vi "OFDM TX.vi"(1 "Samples/Symbol":i32, 2 "Waveform":waveform(cdb)) -> (0 "TX Signal":waveform(cdb))   [LabVIEW 2018]
panel:
  out "size(s)":i32
  out "Waveform w/ Center Freq":dbl[](graph)
  # "Note: Amplitude spikes at start/end of a symbol, reason unknown.\nMay be addressed with QAM Windowing?"
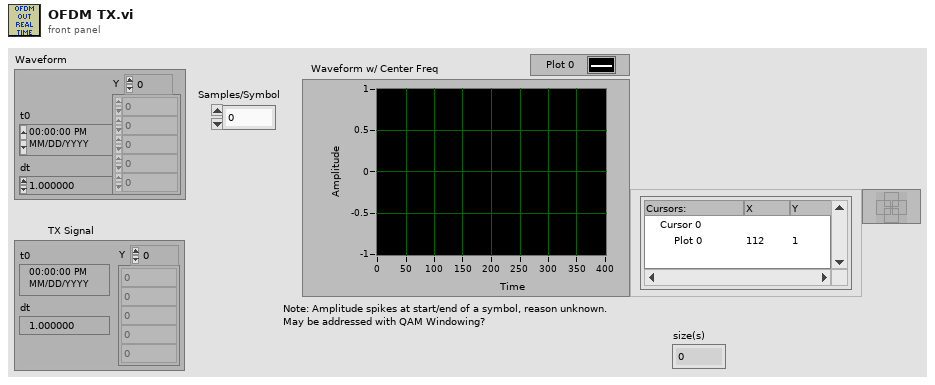
[diagram p1: front panel]
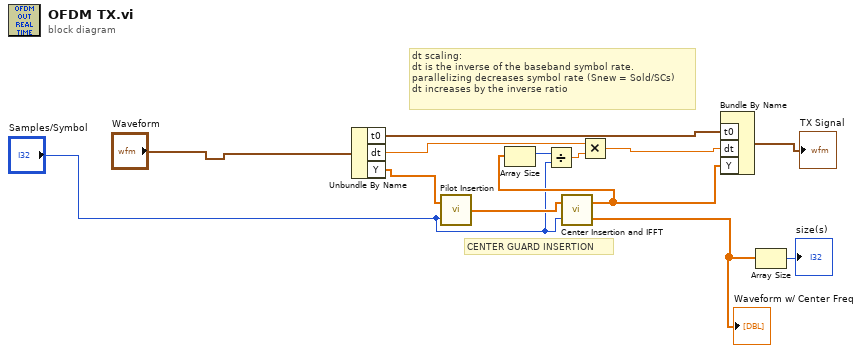
[diagram p0: block diagram]
diagram:
  # "dt scaling:\ndt is the inverse of the baseband symbol rate.\nparallelizing decreases symbol rate (Snew = Sold/SCs)\ndt increases by the inverse ratio"
  # "CENTER GUARD INSERTION"
  n1 = Unbundle By Name("Waveform") -> ("t0"=w11:timestamp, "dt"=w13:dbl, "Y"=w5:cdb[])
  n2 = call "Pilot Insertion.vi"("Samples/Symbol"="Samples/Symbol", "Y(f) in"=w5) -> ("Y(f) out"=w7:cdb[])
  n3 = call "Center Insertion and IFFT.vi"("Samples/Symbol"="Samples/Symbol", "Y(f) in"=w7) -> ("Freq Plot"=w6:dbl[], "Y(t) out"=w4:cdb[])
  "Waveform w/ Center Freq" <- w6
  n4 = Array Size(array=w4) -> (size(s)=w3:i32)
  n5 = Divide(x=w3, y="Samples/Symbol") -> (x/y=w2:dbl)
  n6 = Multiply(x=w13, y=w2) -> (x*y=w10:dbl)
  n7 = Bundle By Name("t0"=w11, "dt"=w10, "Y"=w4) -> (→"TX Signal":waveform(cdb))  [unwired: 1 in]
  n8 = Array Size(array=w6) -> (size(s)=→"size(s)":i32)
